vi "Main_reg.vi"() -> ()   [LabVIEW 2019]
uses:
  _ctrl/create-rw-close.ctl
  _ctrl/rw.ctl
  _ctrl/BP4610_cmd.ctl
  common/load-save_param.ctl
  q-action_reg.ctl
  common/cmd_ui.ctl
  _ctrl/DSP_action.ctl
  _ctrl/Testing-info.ctl
  _ctrl/start.ctl
  Devices/NI Board/cDAQ-9269 AO/AO_q-data.ctl
  sequence_single.ctl
  SubVIs/common/Sample Check.ctl
  Setting_reg.ctl
  Breakdown-Spec.ctl
  Data_reg.ctl
  common/state-machine_result.ctl
  _ctrl/Error list.ctl
panel:
  out "number":u32
  out "n":i32
  out "error cluster 2":T1
  in  "Result data":T2={"NG OK"=TRUE, "Data int"=0, "Daa dbl"=0.0, "Result"=""}
  in  "대기":bool
  in  "status":string
  in  "Tab Control":T3
  out "Pre Charge Relay 2":T4
  out "Pre Charge Relay 6":T4
  out "Pre Charge Relay 5":T4
  out "Pre Charge Relay 4":T4
  out "Pre Charge Relay 3":T4
  out "Pre Charge Relay 1":T4
  out "wfm 6":dbl[](graph)
  out "wfm 5":dbl[](graph)
  out "wfm 4":dbl[](graph)
  out "wfm 3":dbl[](graph)
  out "wfm 2":dbl[](graph)
  out "wfm 1":dbl[](graph)
  out "현재 채널":u8
  out "진행율_채널 %":u8(slide) scale=0.0..100.0
  in  "파일 생성 주기[N]":dbl
  in  "Reg TestSpecs":T6 {"출력단 특성전류 Irms[mA]  Min" format="%#.2f"; "출력단 특성 전류 Irms[mA]  Max" format="%#.2f"; "출력단 단선 Irms[mA](이하)" format="%#.2f"; "제어단 특성 전류 Irms[mA] Min" format="%#.2f"; "제어단 특성 전류 Irms[mA] Max" format="%#.2f"; "제어단 단선 Irms[mA](이하)" format="%#.2f"}
  in  "Test Config":T7
  in  "저장 경로":path
  in  "시험명":string
  out "진행율_전체 %":u8(slide) scale=0.0..100.0
  out "Test Sequence":string
  in  "그래프":bool
  in  "Main":bool
  in  "TestStop":bool
  in  "TestStart":bool
  in  "TestReset":bool
  in  "시험세팅":bool
  in  "Exit":bool
  # "Pre Charge Relay #1"
  # "Pre Charge Relay #4"
  # "Pre Charge Relay #2"
  # "Pre Charge Relay #5"
  # "Pre Charge Relay #3"
  # "Pre Charge Relay #6"
  # "제어단"
  # "출력단"
  # "온도기준"
  # "Highpower"
  # "Control"
  # "Pre Charge Relay 내구시험 (저항부하)"
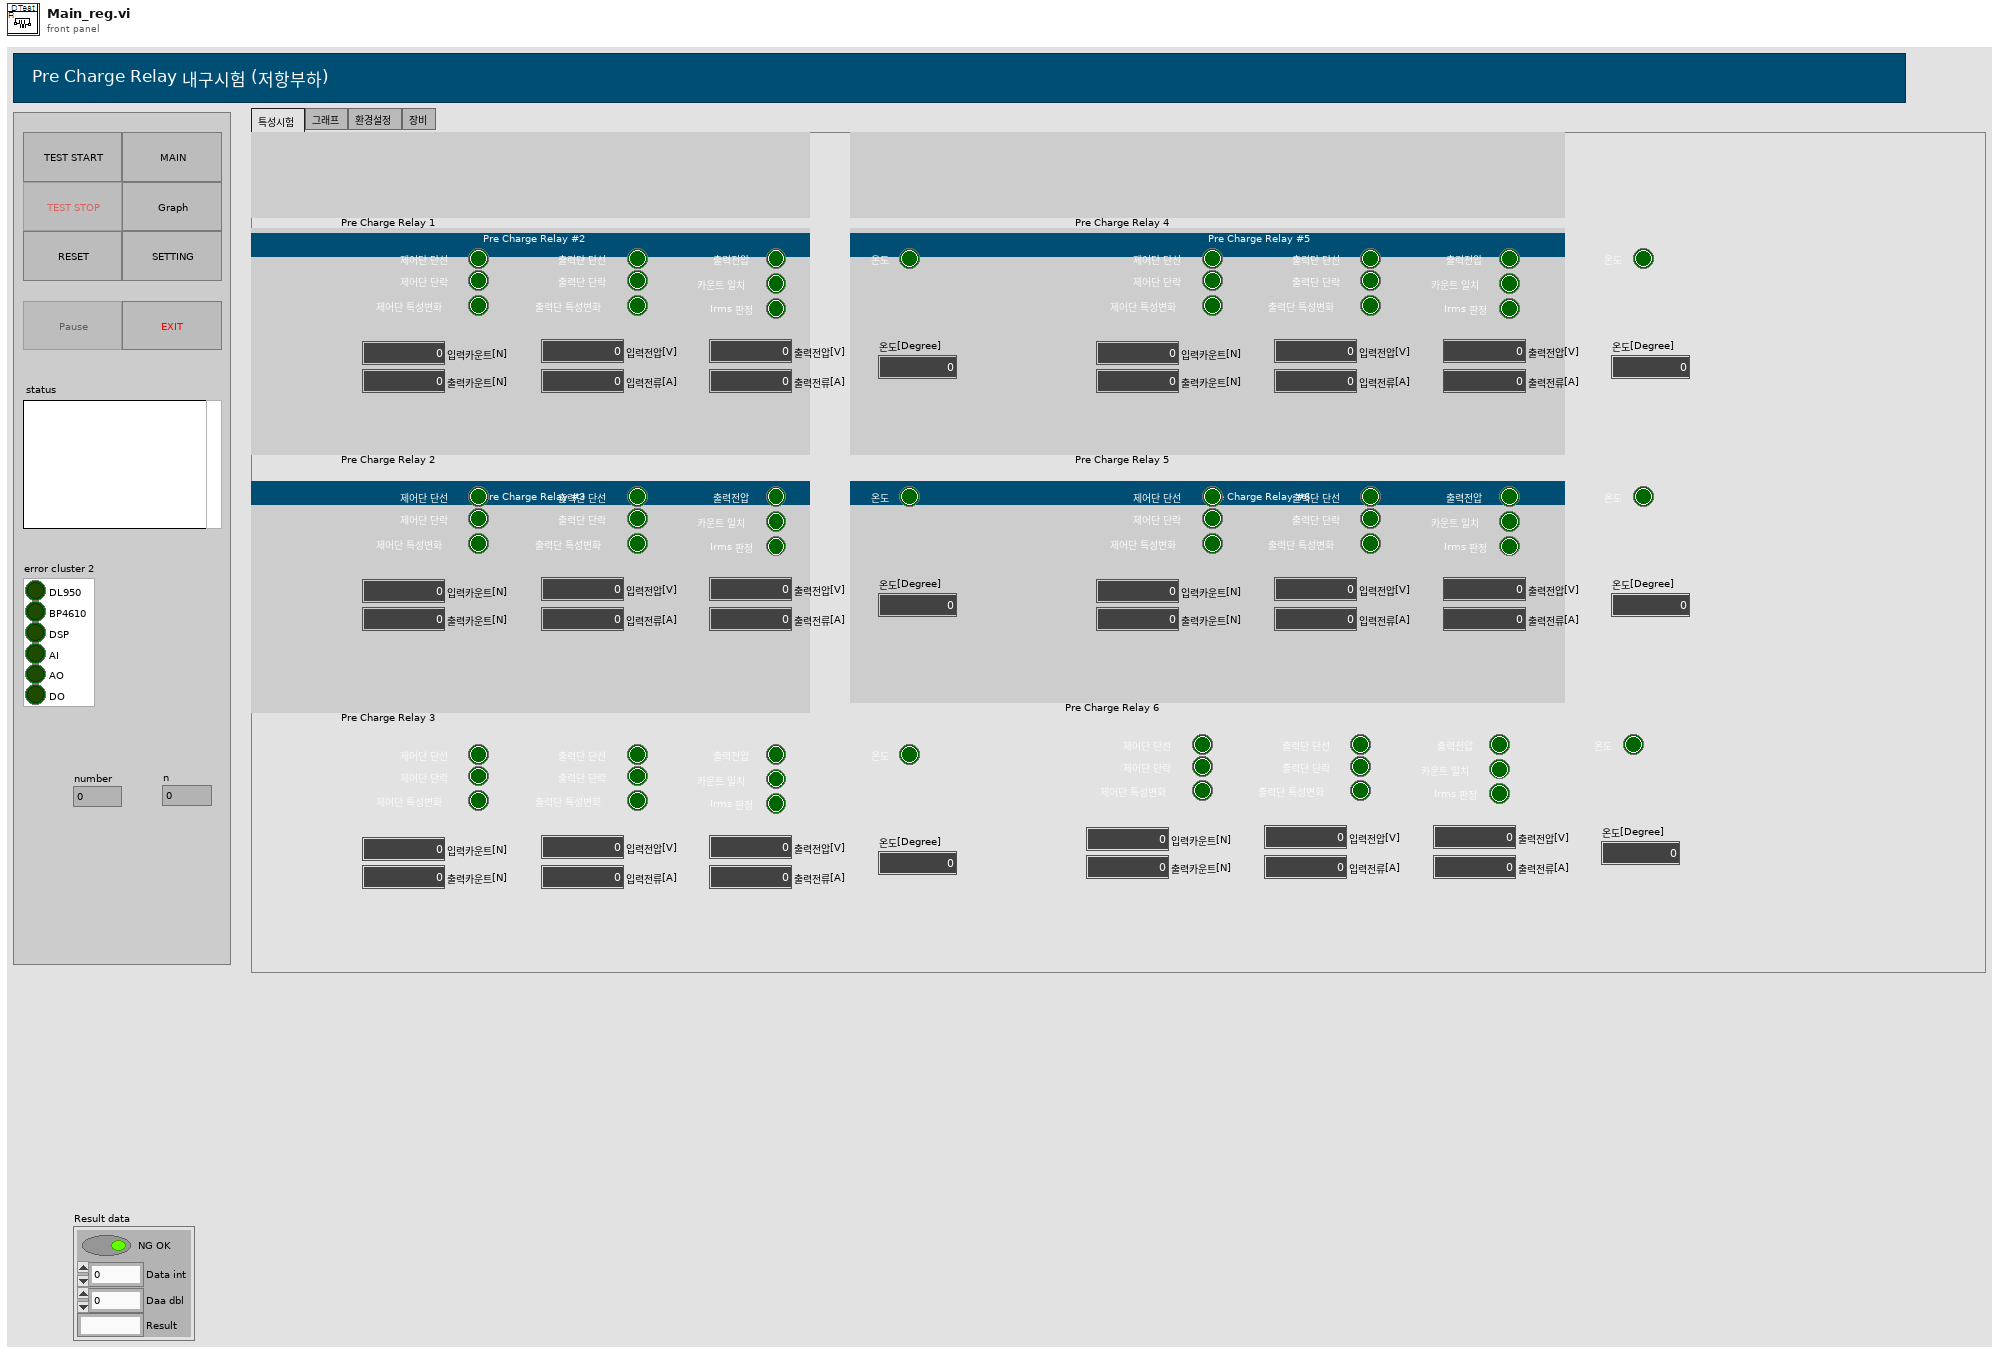
[diagram p1: front panel]
types:
  T1 = typedef "Error list.ctl" = cluster{"DL950":bool, "BP4610":bool, "DSP":bool, "AI":bool, "AO":bool, "DO":bool}
  T2 = typedef "state-machine_result.ctl" = cluster{"NG OK":bool, "Data int":i32, "Daa dbl":dbl, "Result":string}
  T3 = typedef "Tap_내구시험.ctl" = enum32{"특성시험", "그래프", "환경설정", "장비"}
  T4 = typedef "Data_reg.ctl" = cluster{"입력카운트[N]":dbl, "출력카운트[N]":dbl, "입력전압[V]":dbl, "입력전류[A]":dbl, "출력전압[V]":dbl, "출력전류[A]":dbl, "제어단 단선":T5, "제어단 단락":T5, "제어단 특성변화":T5, "출력단 단선":T5, "출력단 단락":T5, "출력단 특성변화":T5, "카운트 일치":T5, "Irms 판정":T5, "출력전압":T5, "온도":T5, "온도[Degree]":dbl}
  T5 = typedef "Sample Check.ctl" = enum32{"idle", "OK", "NG", "Test"}
  T6 = typedef "Breakdown-Spec.ctl" = cluster{"제어단 단선 Irms[mA](이하)":dbl, "제어단 특성 전류 Irms[mA] Max":dbl, "제어단 특성 전류 Irms[mA] Min":dbl, "출력단 단선 Irms[mA](이하)":dbl, "출력단 특성 전류 Irms[mA]  Max":dbl, "출력단 특성전류 Irms[mA]  Min":dbl, "온도[degree]":dbl}
  T7 = typedef "Setting_reg.ctl" = cluster{"제어 전압[V]":dbl, "출력전압[V]":dbl, "전류[A]":dbl, "출력전류[A]":dbl, "ON[초]":dbl, "OFF[초]":dbl, "Irms 허용치 from ":dbl, "Irms 허용치 to":dbl, "AO Delay ms":u32, "Log":path, "result":path}
  T8 = typedef "rw.ctl" = enum16{"read", "write"}
  T9 = typedef "system-status_내구.ctl" = enum16{"Initial", "Update", "Clear"}
  T10 = typedef "create-rw-close.ctl" = enum16{"create", "write", "read", "delete", "close"}
  T11 = typedef "q-action_reg.ctl" = enum16{"Test-ini", "BP4610-on", "Pause", "Test-start", "Group-ini", "Ch-select", "Relay-on", "DSP-on", "DL950-start", "AO-start", "AO-delay", "Delay", "DL950-stop", "DSP-off", "Relay-off", "Ch-check", "UI-update", "Group-end", "Test-stop", "BP4610-off", "Test-finish", "Test-Manual", "DL950-Manual"}
  T12 = enum16{"Config Save", "Config Load", "LastRUN Save", "LastRUN Load"}
  T13 = typedef "load-save_param.ctl" = enum16{"load", "save"}
  T14 = cluster{"TestStart":refnum<vi>, "TestReset":refnum<vi>, "TestStop":refnum<vi>, "Exit":refnum<vi>, "대기":refnum<vi>, "Main":refnum<vi>, "시험세팅":refnum<vi>, "그래프":refnum<vi>}
  T15 = typedef "BP4610_cmd.ctl" = enum16{"open", "read", "set", "set_seq", "limit", "limit_seq", "output on", "output off", "close"}
  T16 = cluster{"ch 1":bool, "ch 2":bool, "ch 3":bool, "ch 4":bool, "ch 5":bool, "ch 6":bool}
  T17 = typedef "Testing-info.ctl" = cluster{"전체채널수":u8, "현재채널번호":u8, "Irms":dbl, "입력전압":dbl, "입력전류":dbl, "출력전압":dbl, "출력전류":dbl, "온도":dbl, "제어단 단선":bool, "제어단 단락":bool, "제어단 특성변화":bool, "출력단 단선":bool, "출력단 단락":bool, "출력단 특성변화":bool, "출력단 전압":bool, "카운트 일치":bool, "Irms 판정":bool, "온도":bool, "테스트 회수":u32, "TestType":T18, "현재회수":u32, "Ch selection":cluster{"1ch":bool, "2ch":bool, "3ch":bool, "4ch":bool, "5ch":bool, "6ch":bool}, "반복":u32, "Path":path, "파일생성주기":u32, "start time":dbl, "stop time":dbl, "현재반복회수":u32, "NG":cluster{"입출력 카운트":bool, "출력전류RMS":bool}}
  T18 = typedef "sequence_single.ctl" = enum16{"Register", "RC", "B1", "B2", "B3"}
  T19 = typedef "cmd_ui.ctl" = enum16{"초기화", "테스트시작", "테스트정지", "테스트종료"}
  T20 = typedef "DSP_action.ctl" = enum16{"False", "cont", "on", "off", "discont", "protection", "protection_seq", "preread", "level_seq", "level_m", "read", "stop", "exit"}
  T21 = typedef "DSP_action.ctl" = enum16{"False", "cont", "on", "off", "discont", "protection", "preread", "level", "read", "stop", "exit"}
  T22 = typedef "start.ctl" = enum16{"init", "open", "set", "start", "stop", "read", "read_items", "query", "close", "T_single", "reset", "exit"}
  T23 = typedef "AO_q-data.ctl" = enum16{"init", "AO start"}
  T24 = typedef "DSP_config.ctl" = cluster{"Port":refnum<visa-resource-name>, "OVP Level":dbl, "OCP Level":dbl, "Current":dbl, "Voltage":dbl}
  T25 = cluster{"Relay 1":refnum<vi>, "Relay 2":refnum<vi>, "Relay 3":refnum<vi>, "Relay 4":refnum<vi>, "Relay 5":refnum<vi>, "Relay 6":refnum<vi>, "고장진단 기준 값":refnum<vi>, "wfm 1":refnum<vi>, "wfm 3":refnum<vi>, "wfm 2":refnum<vi>, "wfm 4":refnum<vi>, "wfm 5":refnum<vi>, "wfm 6":refnum<vi>, "Tab Control":refnum<vi>}
  T26 = typedef "DL950_wfms.ctl" = cluster{"wfms":waveform(dbl)[], "Waveform_2":cluster{"t0":dbl, "dt":dbl, "Y":dbl[][]}, "items":dbl[][], "da950_array":dbl[]}
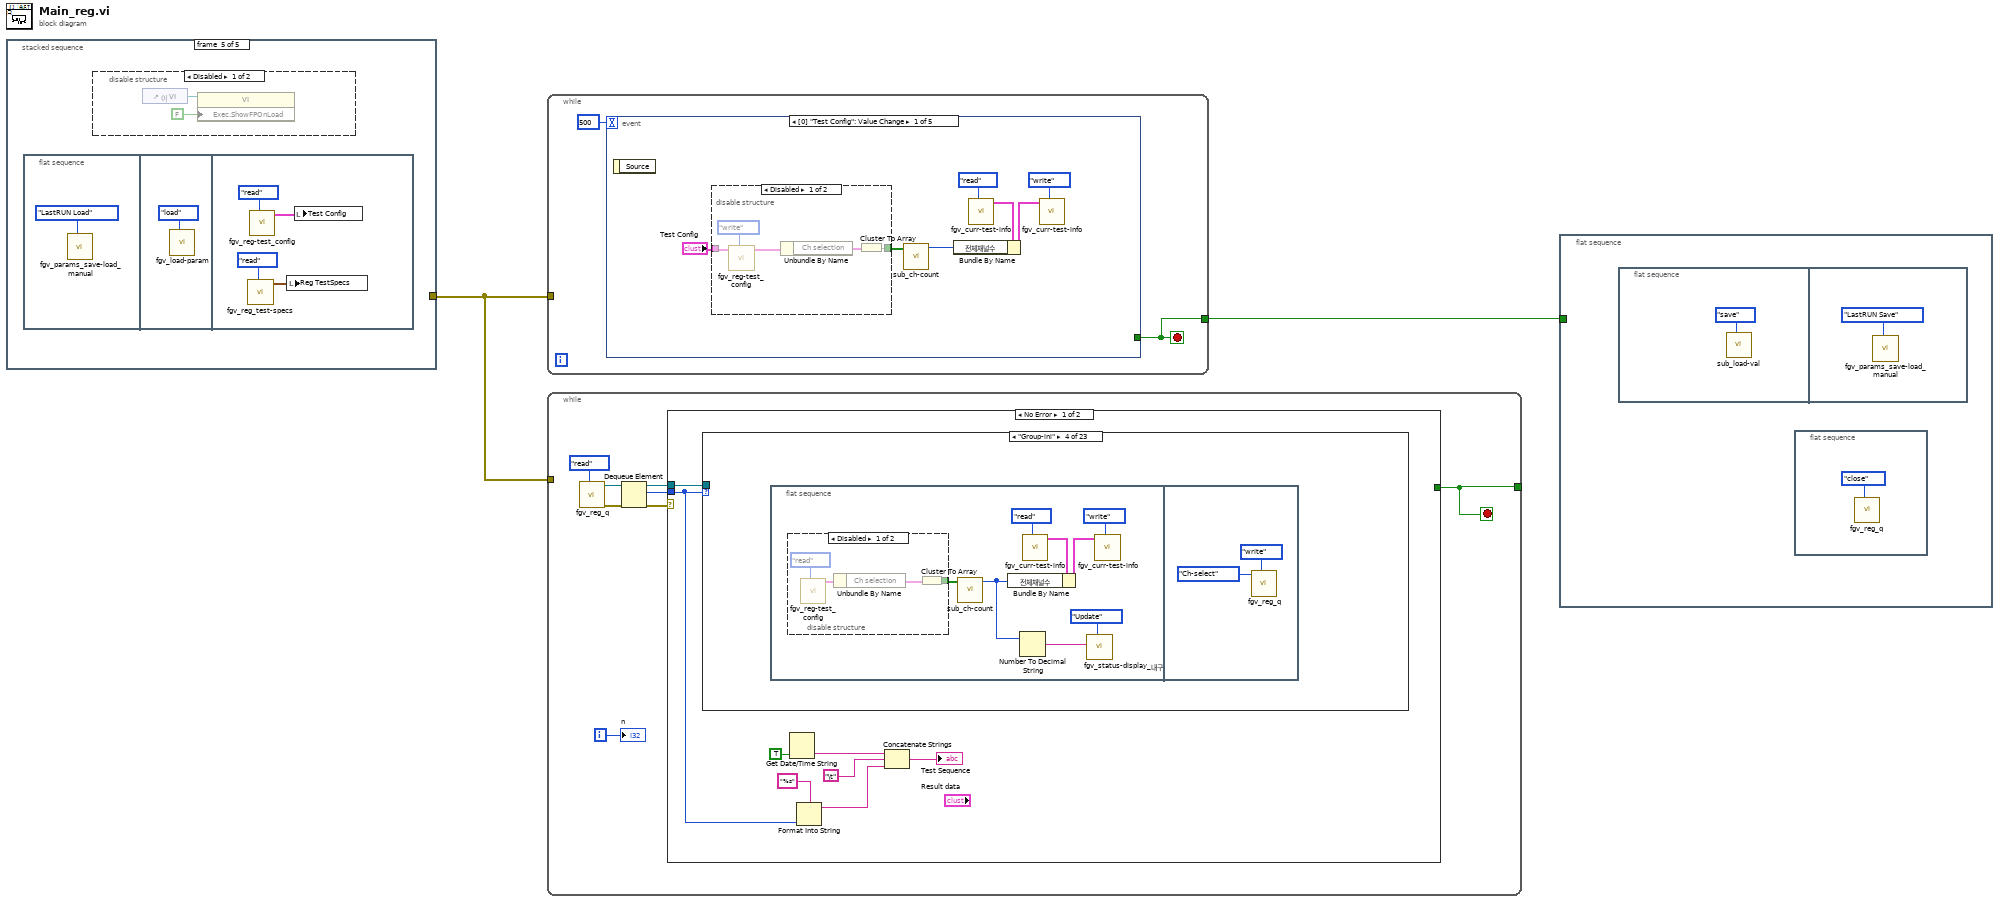
[diagram p0: block diagram]
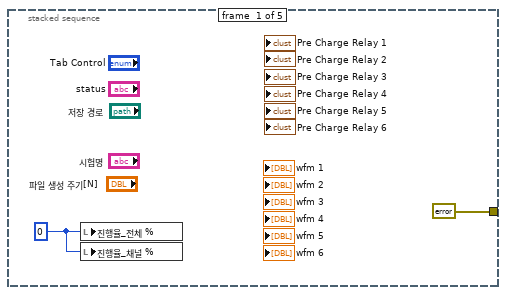
[diagram p2: hidden frame]
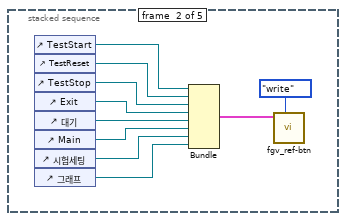
[diagram p3: hidden frame]
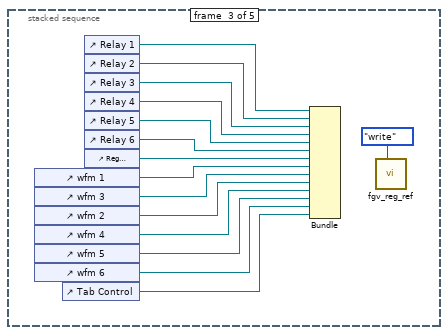
[diagram p4: hidden frame]
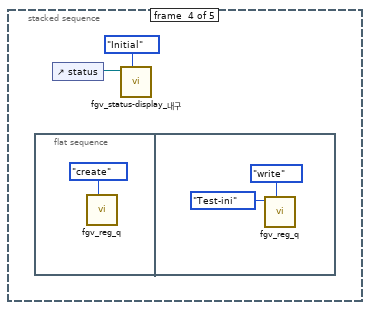
[diagram p5: hidden frame]
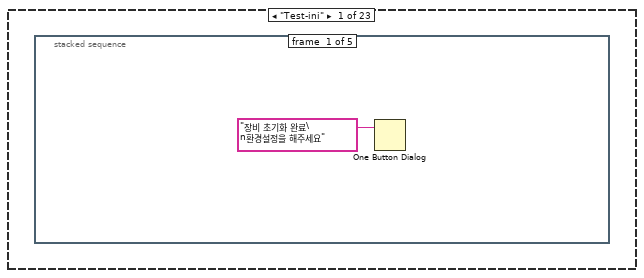
[diagram p7: hidden frame]
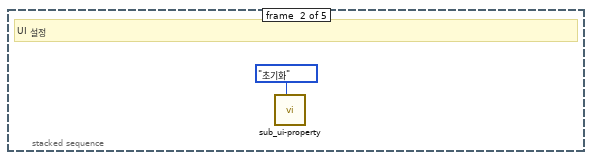
[diagram p8: hidden frame]
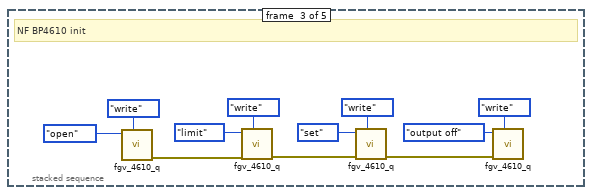
[diagram p9: hidden frame]
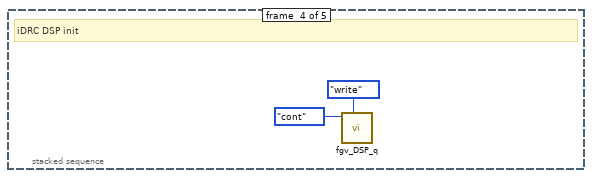
[diagram p10: hidden frame]
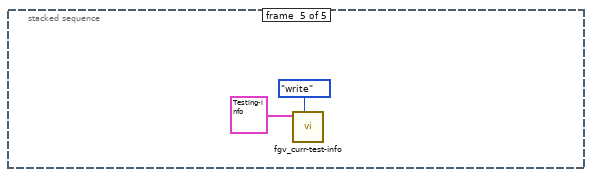
[diagram p11: hidden frame]
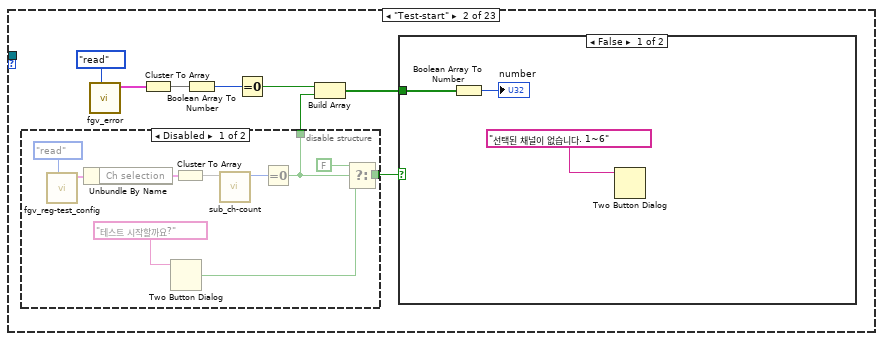
[diagram p12: hidden frame]
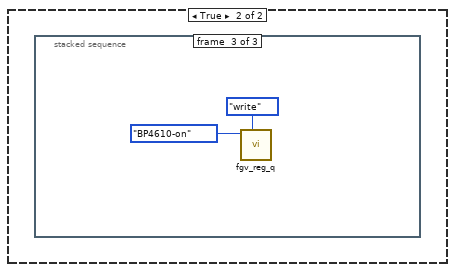
[diagram p14: hidden frame]
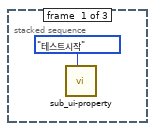
[diagram p15: hidden frame]
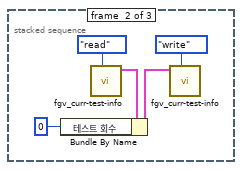
[diagram p16: hidden frame]
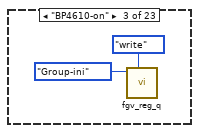
[diagram p17: hidden frame]
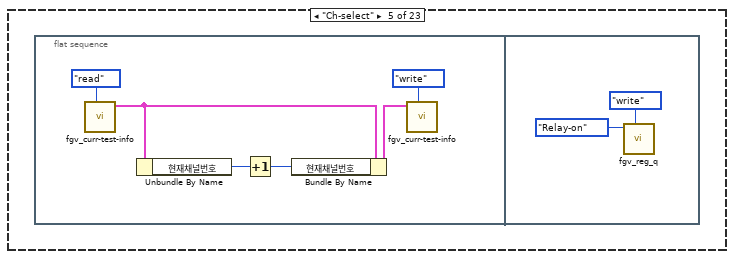
[diagram p19: hidden frame]
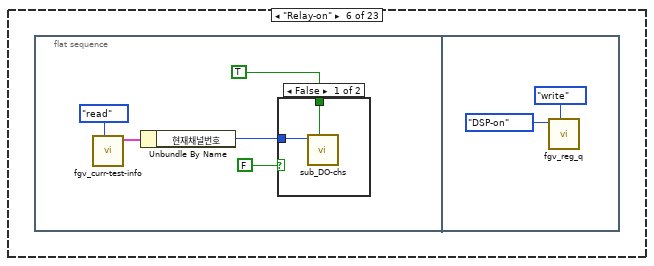
[diagram p20: hidden frame]
diagram:
  n1 = stacked-sequence {
    tunnel: [errorcluster {"status"=FALSE, "code"=0, "source"=""} ("에러 입력(에러 없음)") _ _ _ _] -> w2
    frame #0 {
      w3 = u8 0 ("진행율_전체 %")
      n2 = local write "진행율_전체 %"(w3) -> ()
      n3 = local write "진행율_채널 %"(w3) -> ()
    }
    frame #1 {
      n4 = control-ref of="TestStart"() -> (w14:refnum<vi>)
      n5 = control-ref of="TestReset"() -> (w13:refnum<vi>)
      n6 = control-ref of="TestStop"() -> (w12:refnum<vi>)
      n7 = control-ref of="Exit"() -> (w11:refnum<vi>)
      n8 = control-ref of="대기"() -> (w10:refnum<vi>)
      n9 = control-ref of="Main"() -> (w9:refnum<vi>)
      n10 = control-ref of="시험세팅"() -> (w8:refnum<vi>)
      n11 = control-ref of="그래프"() -> (w7:refnum<vi>)
      n12 = Bundle("TestStart"=w14, "TestReset"=w13, "TestStop"=w12, "Exit"=w11, "대기"=w10, "Main"=w9, "시험세팅"=w8, "그래프"=w7) -> (w6:T14)  [unwired: 1 in]
      n13 = call "fgv_ref-btn.vi"("cmd"=rw."write", "ref"=w6) -> ()  [unwired: 9 in, 1 out]
    }
    frame #2 {
      n14 = control-ref of="wfm 1"() -> (w21:refnum<vi>)
      n15 = control-ref of="wfm 3"() -> (w20:refnum<vi>)
      n16 = control-ref of="wfm 2"() -> (w19:refnum<vi>)
      n17 = control-ref of="wfm 4"() -> (w18:refnum<vi>)
      n18 = control-ref of="wfm 5"() -> (w17:refnum<vi>)
      n19 = control-ref of="wfm 6"() -> (w16:refnum<vi>)
      n20 = control-ref of="Tab Control"() -> (w15:refnum<vi>)
      n21 = control-ref of="Relay 1"() -> (w28:refnum<vi>)
      n22 = control-ref of="Relay 2"() -> (w27:refnum<vi>)
      n23 = control-ref of="Relay 3"() -> (w26:refnum<vi>)
      n24 = control-ref of="Relay 4"() -> (w25:refnum<vi>)
      n25 = control-ref of="Relay 5"() -> (w24:refnum<vi>)
      n26 = control-ref of="Relay 6"() -> (w23:refnum<vi>)
      n27 = control-ref of="Reg TestSpecs"() -> (w22:refnum<vi>)
      n28 = Bundle("Relay 1"=w28, "Relay 2"=w27, "Relay 3"=w26, "Relay 4"=w25, "Relay 5"=w24, "Relay 6"=w23, "Reg TestSpecs"=w22, "wfm 1"=w21, "wfm 3"=w20, "wfm 2"=w19, "wfm 4"=w18, "wfm 5"=w17, "wfm 6"=w16, "Tab Control"=w15) -> ()  [unwired: 1 in, 1 out]
      n29 = call "fgv_reg_ref.vi"("cmd"=rw."write") -> ()  [unwired: 10 in, 1 out]
    }
    frame #3 {
      n30 = flat-sequence {
        frame #0 {
          n31 = call "fgv_reg_q.vi"("cmd"=create-rw-close."create") -> ()  [unwired: 9 in, 2 out]
        }
        frame #1 {
          n32 = call "fgv_reg_q.vi"("cmd"=create-rw-close."write", "action"=q-action_reg."Test-ini") -> ()  [unwired: 8 in, 2 out]
        }
      }
      n33 = control-ref of="status"() -> (w31:refnum<vi>)
      n34 = call "fgv_status-display_내구.vi"("Mode"=system-status_내구."Initial", "System Log"=w31) -> ()  [unwired: 9 in, 1 out]
    }
    frame #4 {
      n35 = flat-sequence {
        frame #0 {
          n36 = call "fgv_params_save-load_manual.vi"("cmd"=T12."LastRUN Load") -> ()  [unwired: 9 in, 2 out]
        }
        frame #1 {
          n37 = call "fgv_load-param.vi"("cmd"=load-save_param."load") -> ()  [unwired: 10 in, 1 out]
        }
        frame #2 {
          n38 = call "fgv_reg_test-specs.vi"("cmd"=rw."read") -> ("고장진단 기준 값 2"=w39:T6)  [unwired: 10 in]
          n39 = call "fgv_reg-test_config.vi"("cmd"=rw."read") -> ("TestConfig out"=w41:T7)  [unwired: 10 in]
          n40 = local write "Reg TestSpecs"(w39) -> ()
          n41 = local write "Test Config"(w41) -> ()
        }
      }
      n42 = disable-structure shown="Disabled" {
        frame Disabled {
          n43 = control-ref of="이 VI"() -> (w36:refnum<vi>)
          n44 = property class="VI"(reference=w36, "Exec.ShowFPOnLoad"=FALSE ("실행:로드 시 프런트패널 보이기")) -> ()  [unwired: 1 in, 2 out]
        }
        frame Enabled {
        }
      }
    }
  }
  n45 = while {
    tunnel: w2 -> [_]
    tunnel: [w44] -> w1
    stop <- w44 stop-if-true
    n46 = event shown="[0] \"Test Config\": Value Change" {
      selector: _ -> [_ _ _ _ _]
      dyn-events: _ -> [_ _ _ _ _]
      timeout: 500 -> [_ _ _ _ _]
      tunnel: [_ _ _ _ w78] -> w44
      event Value Change {
        n47 = event-data() -> ()  [unwired: 1 in, 1 out]
        n48 = disable-structure shown="Disabled" {
          disable-tunnel: "Test Config" -> [w56 _]
          disable-tunnel: [w52 _] -> w46
          frame Disabled {
            n49 = call "fgv_reg-test_config.vi"("cmd"=rw."write", "TestConfig"=w56) -> ("TestConfig out"=w54:T7)  [unwired: 9 in]
            n50 = Unbundle By Name(w54) -> ("Ch selection"=w53:T16)
            n51 = Cluster To Array(cluster=w53) -> (array=w52:bool[])
          }
          frame Enabled {
          }
        }
        n52 = call "sub_ch-count.vi"("ch config"=w46) -> ("ch num"=w45:u8)  [unwired: 10 in]
        n53 = call "fgv_curr-test-info.vi"("cmd"=rw."read") -> ("현재테스트 정보 2"=w48:T17)  [unwired: 10 in]
        n54 = Bundle By Name(cluster=w48, "전체채널수"=w45) -> (w47:T17)
        n55 = call "fgv_curr-test-info.vi"("cmd"=rw."write", "현재테스트 정보"=w47) -> ()  [unwired: 9 in, 1 out]
      }
      event Timeout {
        n56 = event-data() -> ()  [unwired: 1 in, 1 out]
        n57 = stacked-sequence {
          frame #0 {
            n58 = call "fgv_curr-test-info.vi"("cmd"=rw."read") -> ("현재테스트 정보 2"=w65:T17)  [unwired: 10 in]
            n59 = Unbundle By Name(w65) -> ("전체채널수"=w64:u8, "현재채널번호"=w57:u8)  [unwired: 1 out]
            "현재 채널" <- w57
            n60 = Divide(x=w57, y=w64) -> (x/y=w63:dbl)
            n61 = Multiply(x=w63, y=100.0) -> (x*y=w60:dbl)
            n62 = Not Equal?(x=w60, y=w60) -> (x != y?=w61:bool)
            n63 = Select(t=0.0, s=w61, f=w60) -> (s? t:f=→"진행율_채널 %":dbl)
          }
          frame #1 {
            n64 = call "fgv_error.vi"("cmd"=rw."read") -> ("error cluster 2"=→"error cluster 2":T1)  [unwired: 10 in]
          }
        }
      }
      event Value Change {
        n65 = event-data() -> ()  [unwired: 1 in, 2 out]
        n66 = call "fgv_reg_test-specs.vi"("cmd"=rw."write", "고장진단 기준 값"="Reg TestSpecs") -> ()  [unwired: 9 in, 1 out]
      }
      event "시험세팅", "Main", "그래프": Value Change {
        n67 = event-data() -> ("CtlRef"=w73:refnum<vi>)  [unwired: 1 in]
        n68 = property class="Bool"(reference=w73) -> ("Label.Text"=w72:string)  [unwired: 1 in, 2 out]
        n69 = case shown="\"시험세팅\"" w72 {
          tunnel: [Tap_내구시험."특성시험" ("Tab Control") Tap_내구시험."환경설정" ("Tab Control") Tap_내구시험."특성시험" ("Tab Control") Tap_내구시험."그래프" ("Tab Control")] -> w71
          frame "False", Default {
          }
          frame "시험세팅" {
          }
          frame "Main" {
          }
          frame "그래프" {
          }
        }
        n70 = local write "Tab Control"(w71) -> ()
      }
      event "TestReset", "TestStop", "TestStart", "Exit": Value Change {
        n71 = event-data() -> ("CtlRef"=w80:refnum<vi>)  [unwired: 1 in]
        n72 = property class="Bool"(reference=w80) -> ("Label.Text"=w79:string)  [unwired: 1 in, 2 out]
        n73 = case shown="\"TestStop\"" w79 {
          tunnel: [_ _ _ "Exit" _] -> w78
          frame "거짓", Default {
          }
          frame "TestStart" {
            n74 = call "fgv_reg_q.vi"("cmd"=create-rw-close."write", "action"=q-action_reg."Test-start") -> ()  [unwired: 8 in, 2 out]
          }
          frame "TestReset" {
            n75 = call "fgv_reg_q.vi"("cmd"=create-rw-close."write", "action"=q-action_reg."Test-stop") -> ("error out"=w83:errorcluster)  [unwired: 8 in, 1 out]
            n76 = call "fgv_reg_q.vi"("cmd"=create-rw-close."write", "error in"=w83, "action"=q-action_reg."Test-ini") -> ()  [unwired: 7 in, 2 out]
          }
          frame "Exit" {
            n77 = call "fgv_4610_q.vi"("cmd"=create-rw-close."write", "action"=BP4610_cmd."output off") -> ()  [unwired: 8 in, 2 out]
          }
          frame "TestStop" {
            n78 = call "fgv_reg_q.vi"("cmd"=create-rw-close."read") -> ("error out"=w91:errorcluster, "queue out"=w92:refnum<queue>)  [unwired: 9 in]
            n79 = Flush Queue(queue=w92, error in (no error)=w91) -> ()  [unwired: 3 out]
          }
        }
      }
    }
  }
  n80 = while {
    tunnel: [w97] -> _
    tunnel: w2 -> [_]
    i -> [w95]
    stop <- w97 stop-if-true
    n81 = call "fgv_reg_q.vi"("cmd"=create-rw-close."read") -> ("error out"=w98:errorcluster, "queue out"=w94:refnum<queue>)  [unwired: 9 in]
    n82 = Dequeue Element(queue=w94, error in (no error)=w98) -> (queue out=w96:refnum<queue>, element=w100:T11, error out=w101:errorcluster)  [unwired: 1 in, 1 out]
    n83 = case shown="No Error" w101 {
      tunnel: w100 -> [w108 _]
      tunnel: [_ TRUE] -> w97
      tunnel: w96 -> [w109 _]
      frame No Error {
        n84 = case shown="\"Group-ini\"" w108 {
          tunnel: w109 -> [_ _ _ _ _ _ _ _ _ _ _ _ _ _ _ _ _ w288 _ _ _ _ _]
          frame "Test-ini" {
            n85 = stacked-sequence {
              frame #0 {
                n86 = One Button Dialog(message="장비 초기화 완료\n환경설정을 해주세요" ("메시지")) -> ()  [unwired: 1 in, 1 out]
              }
              frame #1 {
                # "UI 설정"
                n87 = call "sub_ui-property.vi"("cmd"=cmd_ui."초기화") -> ()  [unwired: 11 in]
              }
              frame #2 {
                # "NF BP4610 init"
                n88 = call "fgv_4610_q.vi"("cmd"=create-rw-close."write", "action"=BP4610_cmd."open") -> ("error out"=w118:errorcluster)  [unwired: 8 in, 1 out]
                n89 = call "fgv_4610_q.vi"("cmd"=create-rw-close."write", "error in"=w118, "action"=BP4610_cmd."limit") -> ("error out"=w113:errorcluster)  [unwired: 7 in, 1 out]
                n90 = call "fgv_4610_q.vi"("cmd"=create-rw-close."write", "error in"=w113, "action"=BP4610_cmd."set") -> ("error out"=w112:errorcluster)  [unwired: 7 in, 1 out]
                n91 = call "fgv_4610_q.vi"("cmd"=create-rw-close."write", "error in"=w112, "action"=BP4610_cmd."output off") -> ()  [unwired: 7 in, 2 out]
              }
              frame #3 {
                # "iDRC DSP init"
                n92 = call "fgv_DSP_q.vi"("cmd"=create-rw-close."write", "action"=DSP_action."cont") -> ()  [unwired: 8 in, 2 out]
              }
              frame #4 {
                n93 = call "fgv_curr-test-info.vi"("cmd"=rw."write", "현재테스트 정보"=T17 {"전체채널수"=0, "현재채널번호"=0, "Irms"=0.0, "입력전압"=0.0, "입력전류"=0.0, "출력전압"=0.0, "출력전류"=0.0, "온도"=0.0, "제어단 단선"=FALSE, "제어단 단락"=FALSE, "제어단 특성변화"=FALSE, "출력단 단선"=FALSE, "출력단 단락"=FALSE, "출력단 특성변화"=FALSE, "출력단 전압"=FALSE, "카운트 일치"=FALSE, "Irms 판정"=FALSE, "온도"=FALSE, "테스트 회수"=0, "TestType"=enum."Register", "현재회수"=0, "Ch selection"={"1ch"=FALSE, "2ch"=FALSE, "3ch"=FALSE, "4ch"=FALSE, "5ch"=FALSE, "6ch"=FALSE}, "반복"=0, "Path"=path "", "파일생성주기"=0, "start time"=0.0, "stop time"=0.0, "현재반복회수"=0, "NG"={"입출력 카운트"=FALSE, "출력전류RMS"=FALSE}}) -> ()  [unwired: 9 in, 1 out]
              }
            }
          }
          frame "Test-start" {
            n94 = disable-structure shown="Disabled" {
              disable-tunnel: [w136 _] -> w134
              disable-tunnel: [w135 _] -> w129
              frame Disabled {
                n95 = call "fgv_reg-test_config.vi"("cmd"=rw."read") -> ("TestConfig out"=w142:T7)  [unwired: 10 in]
                n96 = Unbundle By Name(w142) -> ("Ch selection"=w141:T16)
                n97 = Two Button Dialog(message="테스트 시작할까요?" ("메시지")) -> (T button?=w138:bool)  [unwired: 2 in]
                n98 = Cluster To Array(cluster=w141) -> (array=w140:bool[])
                n99 = call "sub_ch-count.vi"("ch config"=w140) -> ("ch num"=w139:u8)  [unwired: 10 in]
                n100 = Equal To 0?(x=w139) -> (x = 0?=w135:bool)
                n101 = Select(t=FALSE, s=w135, f=w138) -> (s? t:f=w136:bool)
              }
              frame Enabled {
              }
            }
            n102 = call "fgv_error.vi"("cmd"=rw."read") -> ("error cluster 2"=w132:T1)  [unwired: 10 in]
            n103 = Cluster To Array(cluster=w132) -> (array=w131:bool[])
            n104 = Boolean Array To Number(Boolean array=w131) -> (number=w130:u32)
            n105 = Equal To 0?(x=w130) -> (x = 0?=w128:bool)
            n106 = Build Array(w128, w129) -> (w127:bool[])
            n107 = case shown="False" w134 {
              tunnel: w127 -> [w147 _]
              frame False {
                n108 = Boolean Array To Number(Boolean array=w147) -> (number=→"number":u32)
                n109 = Two Button Dialog(message="선택된 채널이 없습니다. 1~6" ("메시지")) -> ()  [unwired: 2 in, 1 out]
              }
              frame True {
                n110 = stacked-sequence {
                  frame #0 {
                    n111 = call "sub_ui-property.vi"("cmd"=cmd_ui."테스트시작") -> ()  [unwired: 11 in]
                  }
                  frame #1 {
                    n112 = call "fgv_curr-test-info.vi"("cmd"=rw."read") -> ("현재테스트 정보 2"=w149:T17)  [unwired: 10 in]
                    n113 = Bundle By Name(cluster=w149, "테스트 회수"=u8 0 ("현재채널번호")) -> (w151:T17)
                    n114 = call "fgv_curr-test-info.vi"("cmd"=rw."write", "현재테스트 정보"=w151) -> ()  [unwired: 9 in, 1 out]
                  }
                  frame #2 {
                    n115 = call "fgv_reg_q.vi"("cmd"=create-rw-close."write", "action"=q-action_reg."BP4610-on") -> ()  [unwired: 8 in, 2 out]
                  }
                }
              }
            }
          }
          frame "BP4610-on" {
            n116 = call "fgv_reg_q.vi"("cmd"=create-rw-close."write", "action"=q-action_reg."Group-ini") -> ()  [unwired: 8 in, 2 out]
          }
          frame "Group-ini" {
            n117 = flat-sequence {
              frame #0 {
                n118 = disable-structure shown="Disabled" {
                  disable-tunnel: [w166 _] -> w163
                  frame Disabled {
                    n119 = call "fgv_reg-test_config.vi"("cmd"=rw."read") -> ("TestConfig out"=w168:T7)  [unwired: 10 in]
                    n120 = Unbundle By Name(w168) -> ("Ch selection"=w167:T16)
                    n121 = Cluster To Array(cluster=w167) -> (array=w166:bool[])
                  }
                  frame Enabled {
                  }
                }
                n122 = call "sub_ch-count.vi"("ch config"=w163) -> ("ch num"=w158:u8)  [unwired: 10 in]
                n123 = Number To Decimal String(number=w158) -> (decimal integer string=w159:string)  [unwired: 1 in]
                n124 = call "fgv_curr-test-info.vi"("cmd"=rw."read") -> ("현재테스트 정보 2"=w162:T17)  [unwired: 10 in]
                n125 = Bundle By Name(cluster=w162, "전체채널수"=w158) -> (w161:T17)
                n126 = call "fgv_status-display_내구.vi"("Mode"=system-status_내구."Update", "title"=w159) -> ()  [unwired: 9 in, 1 out]
                n127 = call "fgv_curr-test-info.vi"("cmd"=rw."write", "현재테스트 정보"=w161) -> ()  [unwired: 9 in, 1 out]
              }
              frame #1 {
                n128 = call "fgv_reg_q.vi"("cmd"=create-rw-close."write", "action"=q-action_reg."Ch-select") -> ()  [unwired: 8 in, 2 out]
              }
            }
          }
          frame "Ch-select" {
            n129 = flat-sequence {
              frame #0 {
                n130 = call "fgv_curr-test-info.vi"("cmd"=rw."read") -> ("현재테스트 정보 2"=w175:T17)  [unwired: 10 in]
                n131 = Unbundle By Name(w175) -> ("현재채널번호"=w173:u8)
                n132 = Increment(x=w173) -> (x+1=w172:u8)
                n133 = Bundle By Name(cluster=w175, "현재채널번호"=w172) -> (w174:T17)
                n134 = call "fgv_curr-test-info.vi"("cmd"=rw."write", "현재테스트 정보"=w174) -> ()  [unwired: 9 in, 1 out]
              }
              frame #1 {
                n135 = call "fgv_reg_q.vi"("cmd"=create-rw-close."write", "action"=q-action_reg."Relay-on") -> ()  [unwired: 8 in, 2 out]
              }
            }
          }
          frame "Relay-on" {
            n136 = flat-sequence {
              frame #0 {
                n137 = call "fgv_curr-test-info.vi"("cmd"=rw."read") -> ("현재테스트 정보 2"=w183:T17)  [unwired: 10 in]
                n138 = Unbundle By Name(w183) -> ("현재채널번호"=w182:u8)
                n139 = case shown="False" FALSE {
                  tunnel: w182 -> [w185 w188]
                  tunnel: TRUE ("onoff") -> [w186 w187]
                  frame False {
                    n140 = call "sub_DO-chs.vi"("onoff"=w186, "ch"=w185) -> ()  [unwired: 9 in, 1 out]
                  }
                  frame True {
                    n141 = call "sub_DO-relay-onoff.vi"("onoff"=w187, "현재채널번호"=w188) -> ()  [unwired: 10 in]
                  }
                }
              }
              frame #1 {
                n142 = call "fgv_reg_q.vi"("cmd"=create-rw-close."write", "action"=q-action_reg."DSP-on") -> ()  [unwired: 8 in, 2 out]
              }
            }
          }
          frame "DSP-on" {
            (unwired) "DL950 start"
            n143 = case shown="True" TRUE {
              tunnel: [_ w195] -> w191
              frame False {
              }
              frame True {
                n144 = flat-sequence {
                  tunnel: [w202] -> w195
                  frame #0 {
                    n145 = call "fgv_DSP_config.vi"("cmd"=rw."read") -> ("DSP1950 Config 2"=w201:T24)  [unwired: 9 in, 1 out]
                    n146 = Bundle By Name(cluster=w201, "Current"=1.0, "Voltage"=6.0) -> (w200:T24)
                    n147 = call "fgv_DSP_config.vi"("cmd"=rw."write", "DSP1950 Config"=w200) -> ()  [unwired: 8 in, 2 out]
                  }
                  frame #1 {
                    n148 = call "fgv_DSP_q.vi"("cmd"=create-rw-close."write", "action"=DSP_action."level") -> ("error out"=w203:errorcluster)  [unwired: 8 in, 1 out]
                    n149 = call "fgv_DSP_q.vi"("cmd"=create-rw-close."write", "error in"=w203, "action"=DSP_action."on") -> ("error out"=w202:errorcluster)  [unwired: 7 in, 1 out]
                  }
                }
              }
            }
            n150 = flat-sequence {
              tunnel: w191 -> [_]
              frame #0 {
                n151 = call "fgv_reg_q.vi"("cmd"=create-rw-close."write", "action"=q-action_reg."DL950-start") -> ()  [unwired: 8 in, 2 out]
              }
            }
          }
          frame "DL950-start" {
            (unwired) "AO start"
            n152 = flat-sequence {
              frame #0 {
                n153 = call "fgv_DL950_q.vi"("cmd"=create-rw-close."write", "data"=start."start") -> ()  [unwired: 8 in, 2 out]
              }
              frame #1 {
                n154 = Wait (ms)(milliseconds to wait=u32 1000 ("대기 시간 (ms)")) -> ()  [unwired: 1 out]
              }
              frame #2 {
                n155 = call "fgv_reg_q.vi"("cmd"=create-rw-close."write", "action"=q-action_reg."AO-start") -> ()  [unwired: 8 in, 2 out]
              }
            }
          }
          frame "AO-start" {
            (unwired) "Delay"
            n156 = call "fgv_AO_q.vi"("cmd"=create-rw-close."write", "data"=AO_q-data."AO start") -> ("error out"=w214:errorcluster)  [unwired: 8 in, 1 out]
            n157 = call "fgv_reg_q.vi"("cmd"=create-rw-close."write", "error in"=w214, "action"=q-action_reg."AO-delay") -> ()  [unwired: 7 in, 2 out]
          }
          frame "AO-delay" {
            (unwired) "DL950 stop"
            n158 = call "fgv_reg-test_config.vi"("cmd"=rw."read") -> ("TestConfig out"=w221:T7)  [unwired: 10 in]
            n159 = Unbundle By Name(w221) -> ("AO Delay ms"=w220:u32)
            n160 = Wait (ms)(milliseconds to wait=w220) -> ()  [unwired: 1 out]
            n161 = call "fgv_reg_q.vi"("cmd"=create-rw-close."write", "action"=q-action_reg."DL950-stop") -> ()  [unwired: 8 in, 2 out]
          }
          frame "DL950-stop" {
            (unwired) "DSP off"
            n162 = call "fgv_DL950_q.vi"("cmd"=create-rw-close."write", "data"=start."stop") -> ("error out"=w225:errorcluster)  [unwired: 8 in, 1 out]
            n163 = call "fgv_DL950_q.vi"("cmd"=create-rw-close."write", "error in"=w225, "data"=start."read") -> ()  [unwired: 7 in, 2 out]
            n164 = call "fgv_reg_q.vi"("cmd"=create-rw-close."write", "action"=q-action_reg."DSP-off") -> ()  [unwired: 8 in, 2 out]
          }
          frame "DSP-off" {
            (unwired) "Relay off"
            n165 = flat-sequence {
              frame #0 {
                n166 = call "fgv_DSP_config.vi"("cmd"=rw."read") -> ("DSP1950 Config 2"=w233:T24)  [unwired: 9 in, 1 out]
                n167 = Bundle By Name(cluster=w233, "Voltage"=0.0, "Current"=0.0) -> (w232:T24)
                n168 = call "fgv_DSP_config.vi"("cmd"=rw."write", "DSP1950 Config"=w232) -> ()  [unwired: 8 in, 2 out]
              }
              frame #1 {
                n169 = call "fgv_DSP_visa.vi"("action"=DSP_action."level") -> ("error out"=w237:errorcluster)  [unwired: 10 in]
                n170 = call "fgv_DSP_visa.vi"("action"=DSP_action."on", "error in"=w237) -> ()  [unwired: 9 in, 1 out]
              }
              frame #2 {
                n171 = Wait (ms)(milliseconds to wait=u32 400 ("대기 시간 (ms)")) -> ()  [unwired: 1 out]
                n172 = call "fgv_reg_q.vi"("cmd"=create-rw-close."write", "action"=q-action_reg."Relay-off") -> ()  [unwired: 8 in, 2 out]
              }
            }
          }
          frame "Relay-off" {
            n173 = flat-sequence {
              frame #0 {
                n174 = call "fgv_curr-test-info.vi"("cmd"=rw."read") -> ("현재테스트 정보 2"=w244:T17)  [unwired: 10 in]
                n175 = Unbundle By Name(w244) -> ("현재채널번호"=w243:u8)
                n176 = call "sub_DO-relay-onoff.vi"("onoff"=FALSE, "현재채널번호"=w243) -> ()  [unwired: 10 in]
              }
              frame #1 {
                n177 = call "fgv_reg_q.vi"("cmd"=create-rw-close."write", "action"=q-action_reg."UI-update") -> ()  [unwired: 8 in, 2 out]
              }
            }
          }
          frame "Delay" {
            (unwired) q-action_reg."Delay" ("action")
          }
          frame "UI-update" {
            (unwired) "채널체크"
            n178 = flat-sequence {
              frame #0 {
                n179 = call "fgv_reg_ref.vi"("cmd"=rw."read") -> ("output cluster 2"=w252:T25)  [unwired: 10 in]
                n180 = call "fgv_DL950_data.vi"("cmd"=rw."read") -> ("DL950 wfm 2"=w254:T26)  [unwired: 9 in, 1 out]
                n181 = Unbundle By Name(w254) -> ("wfms"=w255:waveform(dbl)[])
                n182 = Unbundle By Name(w252) -> ("wfm 1"=w253:refnum<vi>)  [unwired: 1 out]
                n183 = Index Array(array=w255) -> (element=w256:waveform(dbl))  [unwired: 1 in]
                n184 = property class="WFGraph (strict)"(reference=w253, "Value"=w256) -> ()  [unwired: 1 in, 2 out]
              }
            }
            n185 = call "fgv_reg_q.vi"("cmd"=create-rw-close."write", "action"=q-action_reg."Ch-check") -> ()  [unwired: 8 in, 2 out]
          }
          frame "Ch-check" {
            n186 = call "fgv_curr-test-info.vi"("cmd"=rw."read") -> ("현재테스트 정보 2"=w265:T17)  [unwired: 10 in]
            n187 = Unbundle By Name(w265) -> ("전체채널수"=w263:u8, "현재채널번호"=w262:u8)
            n188 = Equal?(x=w263, y=w262) -> (x = y?=w261:bool)
            n189 = case shown="True" w261 {
              frame False {
              }
              frame True {
                n190 = call "fgv_curr-test-info.vi"("cmd"=rw."read") -> ("현재테스트 정보 2"=w268:T17)  [unwired: 10 in]
                n191 = Unbundle By Name(w268) -> ("테스트 회수"=w267:u32)
                n192 = Increment(x=w267) -> (x+1=w266:u32)
                n193 = Bundle By Name(cluster=w268, "현재채널번호"=u8 0, "테스트 회수"=w266) -> (w270:T17)
                n194 = call "fgv_curr-test-info.vi"("cmd"=rw."write", "현재테스트 정보"=w270) -> ()  [unwired: 9 in, 1 out]
              }
            }
            n195 = Select(t=q-action_reg."Group-end" ("action"), s=w261, f=q-action_reg."Ch-select" ("action")) -> (s? t:f=w257:T11)
            n196 = call "fgv_reg_q.vi"("cmd"=create-rw-close."write", "action"=w257) -> ()  [unwired: 8 in, 2 out]
          }
          frame "Group-end" {
            n197 = disable-structure shown="Disabled" {
              disable-tunnel: [w280 _] -> w277
              frame Disabled {
                n198 = call "fgv_reg-test_config.vi"("cmd"=rw."read") -> ("TestConfig out"=w284:T7)  [unwired: 10 in]
                n199 = call "fgv_curr-test-info.vi"("cmd"=rw."read") -> ("현재테스트 정보 2"=w283:T17)  [unwired: 10 in]
                n200 = Unbundle By Name(w284) -> ("시험횟수[N]"=w281:u32)
                n201 = Unbundle By Name(w283) -> ("테스트 회수"=w282:u32)
                n202 = Equal?(x=w281, y=w282) -> (x = y?=w280:bool)
              }
              frame Enabled {
              }
            }
            n203 = Select(t=q-action_reg."BP4610-off" ("action"), s=w277, f=q-action_reg."Group-ini" ("action")) -> (s? t:f=w273:T11)
            n204 = Select(t="테스트종료", s=w277, f="그룹초기화") -> ()  [unwired: 1 out]
            n205 = call "fgv_reg_q.vi"("cmd"=create-rw-close."write", "action"=w273) -> ()  [unwired: 8 in, 2 out]
          }
          frame "Test-stop" {
            n206 = Flush Queue(queue=w288) -> ()  [unwired: 1 in, 3 out]
            n207 = call "sub_ui-property.vi"("cmd"=cmd_ui."테스트종료") -> ()  [unwired: 11 in]
            n208 = flat-sequence {
              frame #0 {
                n209 = for {
                  N: 6 -> [_]
                  tunnel: FALSE ("onoff") -> [w291]
                  i -> [w293]
                  n210 = Increment(x=w293) -> (x+1=w292:i32)
                  n211 = call "sub_DO-relay-onoff.vi"("onoff"=w291, "현재채널번호"=w292) -> ()  [unwired: 10 in]
                }
              }
              frame #1 {
                n212 = call "fgv_reg_q.vi"("cmd"=create-rw-close."write", "action"=q-action_reg."Test-finish") -> ()  [unwired: 8 in, 2 out]
              }
            }
          }
          frame "BP4610-off" {
            n213 = flat-sequence {
              frame #0 {
                n214 = call "fgv_4610_q.vi"("cmd"=create-rw-close."write", "action"=BP4610_cmd."output off") -> ()  [unwired: 8 in, 2 out]
              }
              frame #1 {
                n215 = call "fgv_reg_q.vi"("cmd"=create-rw-close."write", "action"=q-action_reg."Test-stop") -> ()  [unwired: 8 in, 2 out]
              }
            }
          }
          frame "Test-finish" {
            n216 = One Button Dialog(message="테스트 완료" ("메시지")) -> ()  [unwired: 1 in, 1 out]
            n217 = flat-sequence {
              frame #0 {
                n218 = call "sub_ui-property.vi"("cmd"=cmd_ui."테스트종료") -> ()  [unwired: 11 in]
                n219 = call "fgv_curr-test-info.vi"("cmd"=rw."read") -> ("현재테스트 정보 2"=w302:T17)  [unwired: 10 in]
                n220 = Bundle By Name(cluster=w302, "현재채널번호"=u8 0) -> (w304:T17)
                n221 = call "fgv_curr-test-info.vi"("cmd"=rw."write", "현재테스트 정보"=w304) -> ()  [unwired: 9 in, 1 out]
              }
              frame #1 {
              }
            }
          }
          frame "Pause" {
            n222 = Wait (ms)(milliseconds to wait=u32 100 ("대기 시간 (ms)")) -> ()  [unwired: 1 out]
            n223 = Select(t="그룹초기화", s=FALSE, f="대기") -> ()  [unwired: 1 out]
          }
          frame "Test-Manual" {
          }
          frame "DL950-Manual" {
          }
        }
        n224 = Get Date/Time String(want seconds? (F)=TRUE ("초 보이기? (거짓)")) -> (time string=w104:string)  [unwired: 2 in, 1 out]
        n225 = Format Into String(format string="%s" ("포맷 문자열"), w108) -> (resulting string=w102:string)  [unwired: 2 in, 1 out]
        n226 = Concatenate Strings(w104, "\t", w102) -> (→"Test Sequence":string)
      }
      frame Error {
        # "Return true in any case that should stop the loop."
      }
    }
    "n" <- w95
  }
  n227 = flat-sequence {
    tunnel: w1 -> [_]
    frame #0 {
      n228 = flat-sequence {
        frame #0 {
          n229 = call "sub_load-val.vi"("cmd"=enum16{"load", "save"}."save") -> ()  [unwired: 10 in, 1 out]
        }
        frame #1 {
          n230 = call "fgv_params_save-load_manual.vi"("cmd"=T12."LastRUN Save") -> ()  [unwired: 9 in, 2 out]
        }
      }
      n231 = flat-sequence {
        frame #0 {
          n232 = call "fgv_reg_q.vi"("cmd"=create-rw-close."close") -> ()  [unwired: 9 in, 2 out]
        }
      }
    }
  }
